vi "FPposition.vi"(0 "String In":string, 1 "Action":enum16{"Make string", "Decode string"}(ring)) -> (2 "String Out":string, 3 "top":i32, 4 "left":i32)   [LabVIEW 2014]
uses:
  globals/AzCamGlobals.vi
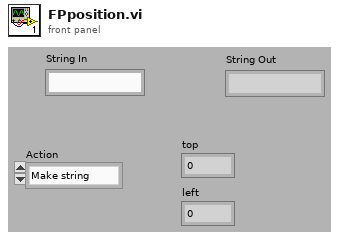
[diagram p1: front panel]
types:
  T1 = typedef "LVRectTypeDef.ctl" = cluster{"Left":i16, "Top":i16, "Right":i16, "Bottom":i16}
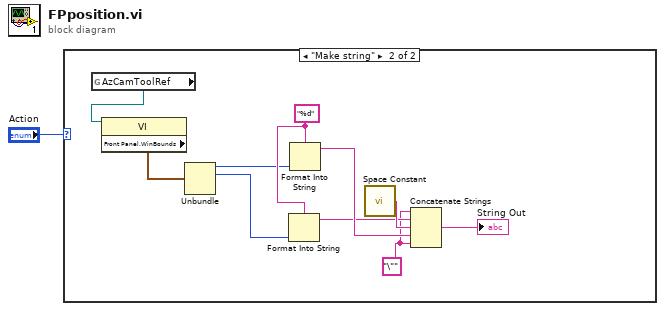
[diagram p0: block diagram]
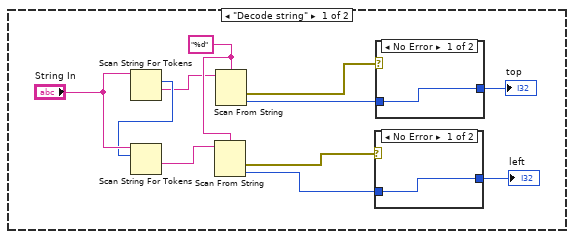
[diagram p2: hidden frame]
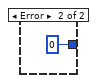
[diagram p3: hidden frame]
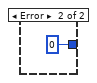
[diagram p4: hidden frame]
diagram:
  n1 = case shown="\"Make string\"" "Action" {
    frame "Decode string" {
      w10 = "%d" ("format string")
      n2 = Scan String For Tokens(9:"String In") -> (1:w9:string, 2:w11:i32)  [unwired: 5 in, 2 out]
      n3 = Scan String For Tokens(8:w11, 9:"String In") -> (1:w8:string)  [unwired: 4 in, 3 out]
      n4 = Scan From String(format string=w10, input string=w8) -> (error out=w2:errorcluster, output 1=w3:i32)  [unwired: 3 in, 2 out]
      n5 = Scan From String(format string=w10, input string=w9) -> (error out=w7:errorcluster, output 1=w5:i32)  [unwired: 3 in, 2 out]
      n6 = case shown="No Error" w2 {
        tunnel: [w13 0] -> w4
        tunnel: w3 -> [w13 _]
        frame No Error {
        }
        frame Error {
        }
      }
      "left" <- w4
      n7 = case shown="No Error" w7 {
        tunnel: [w15 0] -> w6
        tunnel: w5 -> [w15 _]
        frame No Error {
        }
        frame Error {
        }
      }
      "top" <- w6
    }
    frame "Make string" {
      w17 = "\""
      w26 = "%d" ("format string")
      n8 = global read "AzCamGlobals.vi" "AzCamToolRef"() -> (w19:refnum<vi>)
      n9 = property class="VI"(reference=w19) -> ("Front Panel.WinBounds"=w18:T1)  [unwired: 1 in, 2 out]
      n10 = Unbundle(w18) -> ("Left"=w25:i16, "Top"=w24:i16)  [unwired: 2 out]
      n11 = Format Into String(format string=w26, w24) -> (resulting string=w20:string)  [unwired: 2 in, 1 out]
      n12 = Format Into String(format string=w26, w25) -> (resulting string=w21:string)  [unwired: 2 in, 1 out]
      n13 = call <vilib>:"Space Constant.vi"() -> ("String"=w22:string)
      n14 = Concatenate Strings(w17, w20, w22, w21, w17) -> (→"String Out":string)
    }
  }
